vi "setReadOutFreq.vi"(8 "error":errorcluster, 9 "RESReadOutFreq_Hz":i32, 10 "axis [0|1|2]":u8, 11 "connection ID":refnum<k5>) -> (0 "error out":errorcluster, 1 "RESReadOutFreq_Hz_Readback":i32, 2 "axis out":u8, 3 "connection ID out":refnum<k5>)   [LabVIEW 2016, in "AMC_VIs.lvlib"]
doc: "This function reads the frequency for the sensor read out of the RES position on a specific axis\nInputs:\n -- connection string (from connect_TCP.vi)\n -- axis [0|1|2]\n -- Readout Frequency [Hz]\n\nOutputs:\n -- connection ID out\n -- axis out"
uses:
  AMC_VIs.lvlib
panel:
  out "JSON-response":string="{\"jsonrpc\":\"2.0\",\"method\":\"\",\"params\":[5,1.245,true,\"name\"],\"id\":\"1\"}"
  out "JSON request":string
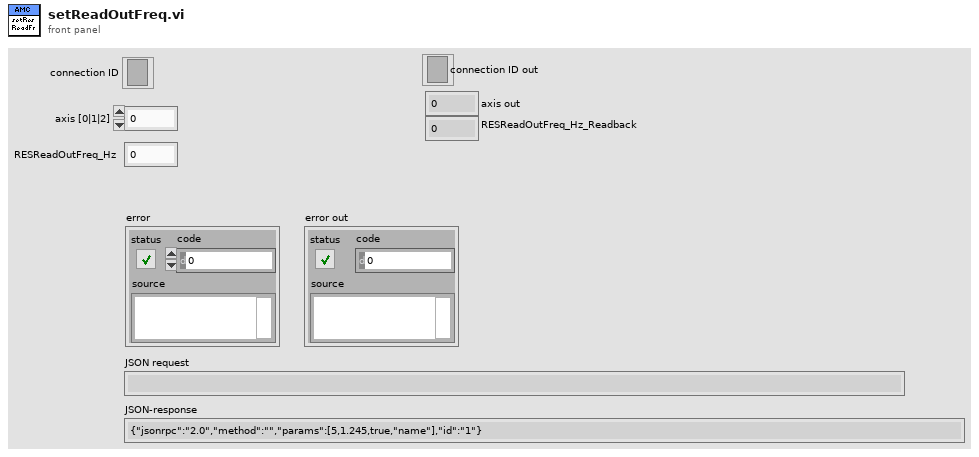
[diagram p1: front panel]
types:
  T1 = cluster{"jsonrpc":string, "method":string, "params":i32[], "id":string, "api":string}
  T2 = cluster{"jsonrpc":string, "result":i32[], "id":string}
  T3 = enum16{"Standard", "Buffered", "CRLF", "Immediate"}
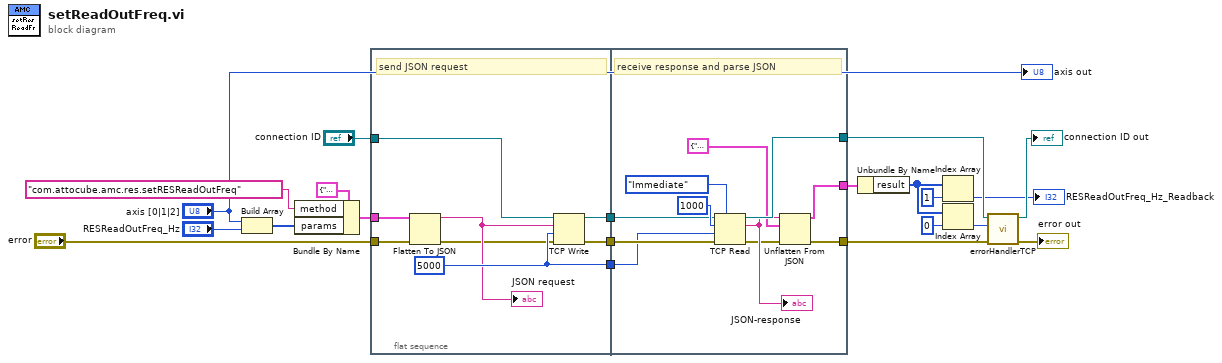
[diagram p0: block diagram]
diagram:
  n1 = Build Array("axis [0|1|2]", "RESReadOutFreq_Hz") -> (w13:i32[])
  n2 = Bundle By Name(cluster=T1 {"jsonrpc"="2.0", "method"="com.attocube.amc.res.setRESReadOutFreq", "params"=[0, 2712], "id"="1", "api"="2"} ("InputParams 2"), "method"="com.attocube.amc.res.setRESReadOutFreq", "params"=w13) -> (w12:T1)
  n3 = flat-sequence {
    tunnel: "connection ID" -> [w29]
    tunnel: [w27] -> w21
    tunnel: [w28] -> w20
    tunnel: "error" -> [w23]
    tunnel: [w26] -> w19
    tunnel: w12 -> [w25]
    tunnel: [w36] -> w4
    tunnel: w21 -> [w38]
    tunnel: w20 -> [w37]
    tunnel: [w32] -> w7
    tunnel: w19 -> [w35]
    tunnel: [w31] -> w11
    frame #0 {
      w26 = 5000 ("timeout ms (25000)")
      # "send JSON request"
      n4 = Flatten To JSON(anything=w25, error in (no error)=w23) -> (JSON string=w24:string, 11:w22:errorcluster)  [unwired: 1 in]
      "JSON request" <- w24
      n5 = TCP Write(connection ID=w29, data in=w24, error in (no error)=w22, 9:w26) -> (connection ID out=w27:refnum<k5>, error out=w28:errorcluster)  [unwired: 1 out]
    }
    frame #1 {
      # "receive response and parse JSON"
      n6 = TCP Read(connection ID=w38, bytes to read=1000, error in (no error)=w37, 7:T3."Immediate" ("mode (standard)"), 9:w35) -> (connection ID out=w36:refnum<k5>, data out=w34:string, error out=w33:errorcluster)
      "JSON-response" <- w34
      n7 = Unflatten From JSON(JSON string=w34, type and defaults=T2 {"jsonrpc"="2.0", "result"=[0, 2712], "id"="1"} ("InputParams 2"), error in (no error)=w33) -> (value=w31:T2, error out=w32:errorcluster)  [unwired: 4 in]
    }
  }
  n8 = Unbundle By Name(w11) -> ("result"=w8:i32[])
  n9 = Index Array(array=w8, index=1) -> (element=→"RESReadOutFreq_Hz_Readback":i32)
  n10 = Index Array(array=w8, index=0) -> (element=w6:i32)
  n11 = call "errorHandlerTCP.vi"("error in"=w7, "error number"=w6, "connection ID"=w4) -> ("error out"=→"error out":errorcluster, "connection ID"=→"connection ID out":refnum<k5>)  [unwired: 7 in]
  "axis out" <- "axis [0|1|2]"
